vi "PRO_Detect Switch Point_V1.vi"(6 "error in (no error)":errorcluster, 8 "Drain!Fill":bool, 9 "Fitler TC":dbl=0.9, 10 "Measure N-1":T2={"Ch A   Ohms"=100.0, " Ch B  Ohms"=100.0, "Level OUt"=3.672222222222213}, 11 "Measure N":T2={"Ch A   Ohms"=100.0, " Ch B  Ohms"=200.0, "Level OUt"=3.699999999999991}) -> (0 "ChB Switch":bool=TRUE, 1 "ChA Switch":bool, 2 "XResult":T1=[{"Switched"=FALSE, "In Range"=TRUE, "Index"=1, "Level OUt"=3.699999999999991, " Ch n Ohms"=100.0, "Drain!Fill"=FALSE}, {"Switched"=TRUE, "In Range"=TRUE, "Index"=2, "Level OUt"=3.699999999999991, " Ch n Ohms"=100.0, "Drain!Fill"=FALSE}], 3 "Measure N out":T2={"Ch A   Ohms"=100.0, " Ch B  Ohms"=200.0, "Level OUt"=3.697222222222213}, 4 "error out":errorcluster)   [LabVIEW 2024]
uses:
  Control Definitions/Def Xresult.ctl
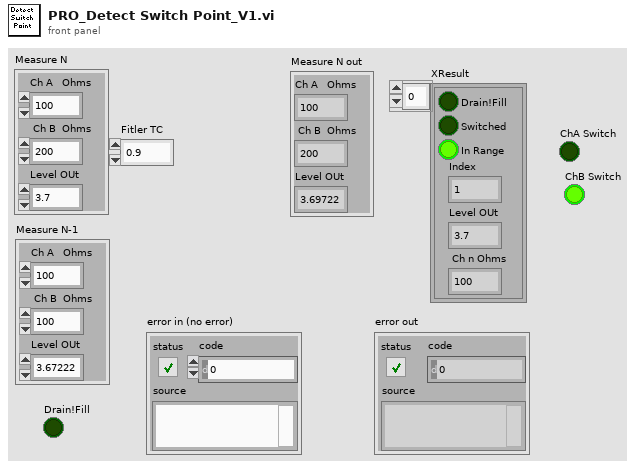
[diagram p1: front panel]
types:
  T1 = typedef "Def Xresult.ctl" = cluster{"Switched":bool, "In Range":bool, "Index":i16, "Level OUt":dbl, " Ch n Ohms":dbl, "Drain!Fill":bool}[]
  T2 = cluster{"Ch A   Ohms":dbl, " Ch B  Ohms":dbl, "Level OUt":dbl}
  T3 = cluster{"XSwitch":bool, "In Range?":bool, "Rindex":i16, "Level OUt":dbl, "Ch A   Ohms":dbl, "Drain!Fill":bool}
  T4 = cluster{"XSwitch":bool, "In Range?":bool, "Rindex":i16, "Level OUt":dbl, " Ch B  Ohms":dbl, "Drain!Fill":bool}
  T5 = cluster{"XSwitch":bool, "In Range?":bool, "Rindex":i16, "Level OUt":dbl, " Ch B  Ohms":dbl, "Drain!Fill":bool}[]
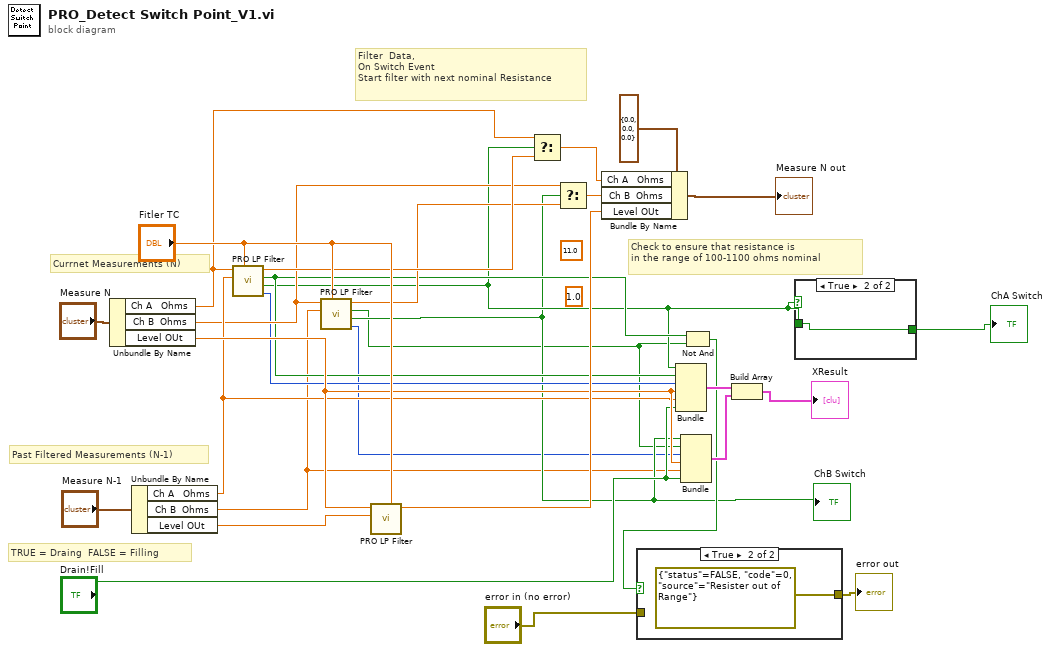
[diagram p0: block diagram]
diagram:
  (unwired) 1.0 ("lower limit")
  (unwired) 11.0 ("upper limit")
  # "TRUE = Draing  FALSE = Filling"
  # "Past Filtered Measurements (N-1)"
  # "Currnet Measurements (N)"
  # "Check to ensure that resistance is \nin the range of 100-1100 ohms nominal"
  # "Filter  Data, \nOn Switch Event\nStart filter with next nominal Resistance"
  n1 = Unbundle By Name("Measure N") -> ("Ch A   Ohms"=w10:dbl, "Ch B  Ohms"=w9:dbl, "Level OUt"=w14:dbl)
  n2 = Unbundle By Name("Measure N-1") -> ("Ch A   Ohms"=w13:dbl, "Ch B  Ohms"=w2:dbl, "Level OUt"=w23:dbl)
  n3 = call "PRO LP Filter.vi"("Fitler TC"="Fitler TC", "In N -1"=w13, "In N"=w10) -> ("Rindex"=w7:i16, "XSwitch"=w6:bool, "In Range?"=w8:bool, "Filtered Out"=w20:dbl)  [unwired: 5 in]
  n4 = call "PRO LP Filter.vi"("Fitler TC"="Fitler TC", "In N -1"=w2, "In N"=w9) -> ("Rindex"=w4:i16, "XSwitch"=w5:bool, "In Range?"=w3:bool, "Filtered Out"=w18:dbl)  [unwired: 5 in]
  "ChB Switch" <- w5
  n5 = call "PRO LP Filter.vi"("Fitler TC"="Fitler TC", "In N -1"=w23, "In N"=w14) -> ("Filtered Out"=w16:dbl)  [unwired: 5 in, 3 out]
  n6 = Select(t=w10, s=w6, f=w20) -> (s? t:f=w19:dbl)
  n7 = Select(t=w9, s=w5, f=w18) -> (s? t:f=w17:dbl)
  n8 = Bundle By Name(cluster=T2 {"Ch A   Ohms"=0.0, " Ch B  Ohms"=0.0, "Level OUt"=0.0} ("Cluster N"), "Ch A   Ohms"=w19, "Ch B  Ohms"=w17, "Level OUt"=w16) -> (→"Measure N out":T2)
  n9 = Bundle("XSwitch"=w6, "In Range?"=w8, "Rindex"=w7, "Level OUt"=w14, "Ch A   Ohms"=w13, "Drain!Fill"="Drain!Fill") -> (w29:T3)  [unwired: 1 in]
  n10 = Bundle("XSwitch"=w5, "In Range?"=w3, "Rindex"=w4, "Level OUt"=w14, "Ch B  Ohms"=w2, "Drain!Fill"="Drain!Fill") -> (w28:T4)  [unwired: 1 in]
  n11 = Not And(1:w3, 2:w8) -> (0:w25:bool)
  n12 = case shown="True" w25 {
    tunnel: "error in (no error)" -> [w31 _]
    tunnel: [w31 errorcluster {"status"=FALSE, "code"=0, "source"="Resister out of Range"} ("error out")] -> w26
    frame False {
    }
    frame True {
    }
  }
  "error out" <- w26
  n13 = Build Array(w29, w28) -> (→"XResult":T5)
  n14 = case shown="True" w6 {
    selector: w6 -> [w33 _]
    tunnel: w6 -> [_ w34]
    tunnel: [w33 w34] -> w1
    frame False {
    }
    frame True {
    }
  }
  "ChA Switch" <- w1
